vi "DE_Initialize State.vi"(6 "DE settings":T1={"population size"=10, "scale factor"=0.9, "crossover probability"=0.95, "bound mapping method"=1, "mutation method"=0, "crossover method"=0} {"crossover method" items=["Uniform", "Exponential"]; "mutation method" items=["Random", "Either Or", "Best", "Target to Best"]; "bound mapping method" items=["None", "Random between Bounds and Values", "Re-Initialize"]}, 8 "error in (no error)":errorcluster, 10 "Bounds":cluster{"Min":dbl[], "Max":dbl[]}, 11 "Init Parameters":dbl[][](array[numeric])) -> (0 "error out":errorcluster, 3 "State":T5)   [LabVIEW 2017, in "NI_AAL_GlobalOptimization.lvlib"]
uses:
  <vilib>/gmath/NI_AAL_GlobalOptimization.lvlib
  <vilib>/gmath/GlobalOptimization.llb/DE_State.ctl
  <vilib>/gmath/GlobalOptimization.llb/DE_Population.ctl
  <vilib>/gmath/GlobalOptimization.llb/DE_Settings.ctl
  <vilib>/gmath/GlobalOptimization.llb/DE_Bound Mapping Method.ctl
  <vilib>/gmath/GlobalOptimization.llb/DE_Mutation Method.ctl
  <vilib>/gmath/GlobalOptimization.llb/DE_Crossover Method.ctl
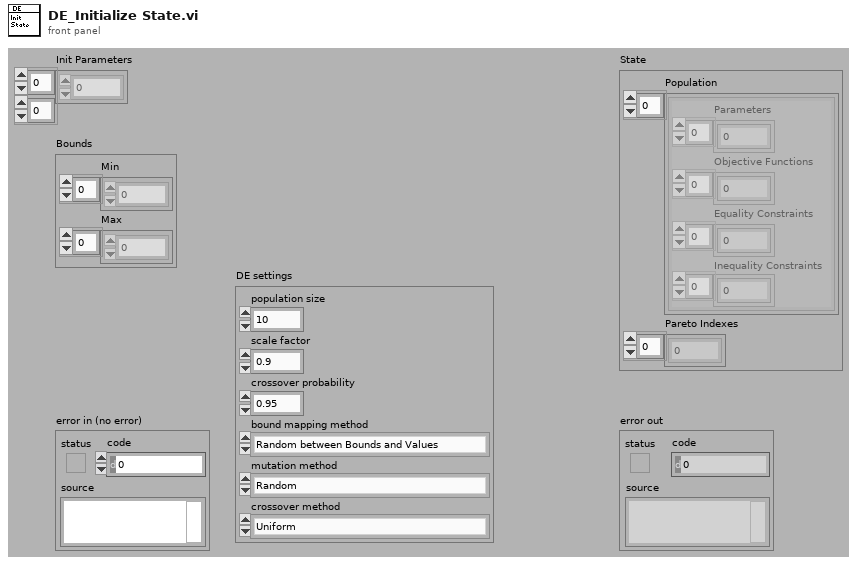
[diagram p1: front panel]
types:
  T1 = typedef "NI_AAL_GlobalOptimization.lvlib/DE_Settings.ctl" = cluster{"population size":i32, "scale factor":dbl, "crossover probability":dbl, "bound mapping method":T2, "mutation method":T3, "crossover method":T4}
  T2 = typedef "NI_AAL_GlobalOptimization.lvlib/DE_Bound Mapping Method.ctl" = u16
  T3 = typedef "NI_AAL_GlobalOptimization.lvlib/DE_Mutation Method.ctl" = u16
  T4 = typedef "NI_AAL_GlobalOptimization.lvlib/DE_Crossover Method.ctl" = u16
  T5 = typedef "NI_AAL_GlobalOptimization.lvlib/DE_State.ctl" = cluster{"Population":T6[], "Pareto Indexes":i32[]}
  T6 = typedef "NI_AAL_GlobalOptimization.lvlib/DE_Population.ctl" = cluster{"Parameters":dbl[], "Objective Functions":dbl[], "Equality Constraints":dbl[], "Inequality Constraints":dbl[]}
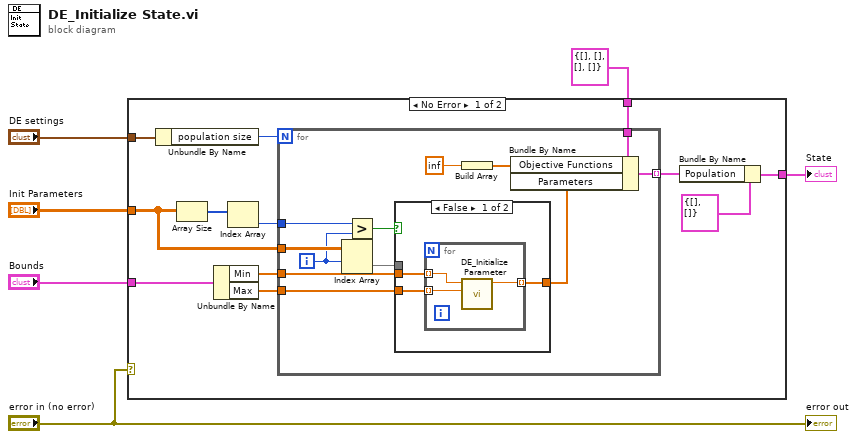
[diagram p0: block diagram]
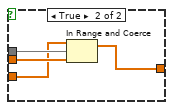
[diagram p2: hidden frame]
diagram:
  n1 = case shown="No Error" "error in (no error)" {
    tunnel: [w18 _] -> w5
    tunnel: "DE settings" -> [w12 _]
    tunnel: "Bounds" -> [w15 _]
    tunnel: T6 {"Parameters"=[], "Objective Functions"=[], "Equality Constraints"=[], "Inequality Constraints"=[]} ("Population") -> [w11 _]
    tunnel: "Init Parameters" -> [w7 _]
    frame No Error {
      n2 = Unbundle By Name(w12) -> ("population size"=w16:i32)
      n3 = Array Size(array=w7) -> (size(s)=w9:i32[])
      n4 = Unbundle By Name(w15) -> ("Min"=w14:dbl[], "Max"=w13:dbl[])
      n5 = Index Array(array=w9) -> (element=w8:i32)  [unwired: 1 in]
      n6 = for {
        N: w16 -> [_]
        tunnel: [w28] -> w17 mode=indexing
        tunnel: w14 -> [w26]
        tunnel: w13 -> [w25]
        tunnel: w11 -> [w24]
        tunnel: w8 -> [w23]
        tunnel: w7 -> [w21]
        i -> [w20]
        n7 = Index Array(array=w21, index (row)=w20) -> (element=w19:dbl[])  [unwired: 1 in]
        n8 = Greater?(x=w23, y=w20) -> (0:w22:bool)
        n9 = case shown="False" w22 {
          tunnel: [w33 w37] -> w30
          tunnel: w26 -> [w32 w39]
          tunnel: w25 -> [w31 w38]
          tunnel: w19 -> [_ w40]
          frame False {
            n10 = for {
              tunnel: [w36] -> w33 mode=indexing
              tunnel: w32 -> [w35] mode=indexing
              tunnel: w31 -> [w34] mode=indexing
              n11 = call <vilib>:"DE_Initialize Parameter.vi"("max bound"=w34, "min bound"=w35) -> ("parameter"=w36:dbl)  [unwired: 9 in]
            }
          }
          frame True {
            n12 = In Range and Coerce(upper limit=w38, x=w40, lower limit=w39) -> (coerced(x)=w37:dbl[])  [unwired: 1 out]
          }
        }
        n13 = Build Array(inf ("Element Data")) -> (w27:dbl[])
        n14 = Bundle By Name(cluster=w24, "Objective Functions"=w27, "Parameters"=w30) -> (w28:T6)
      }
      n15 = Bundle By Name(cluster=T5 {"Population"=[], "Pareto Indexes"=[]} ("State"), "Population"=w17) -> (w18:T5)
    }
    frame Error {
    }
  }
  "State" <- w5
  "error out" <- "error in (no error)"
